vi "Get Metadata.vi"(7 "error in":errorcluster, 9 "measurement control path":path, 10 "measurement plugin service in":refnum<class "Measurement Plugin Service.lvclass">) -> (0 "error out":errorcluster, 2 "metadata value":T2(array[cluster]), 3 "measurement plugin service out":refnum<class "Measurement Plugin Service.lvclass">)   [LabVIEW 2020, in "Measurement Plugin Measurement Server.lvlib"]
uses:
  Measurement Plugin Measurement Server.lvlib
  TypeDefs/Parameter Annotations Entry.ctl
  Measurement Plugin Service/Measurement Plugin Service.lvclass
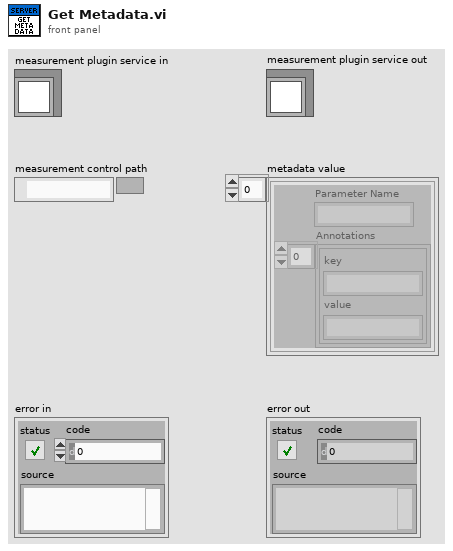
[diagram p1: front panel]
types:
  T1 = typedef "Measurement Plugin Measurement Server.lvlib/Parameter Annotations Entry.ctl" = cluster{"key":string, "value":string}
  T2 = cluster{"Parameter Name":string, "Annotations":T1[]}[]
  T3 = typedef "Measurement Plugin Measurement Server.lvlib/Parameter Type Specialization.ctl" = cluster{"parameter name":string, "type specialization":T4, "annotations":cluster{"key":T5, "value":string}[]}
  T4 = typedef "Measurement Plugin Measurement Server.lvlib/Type Specialization.ctl" = enum16{"none", "pin", "path", "enum", "ioresource"}
  T5 = typedef "Measurement Plugin Measurement Server.lvlib/Type Specialization Key.ctl" = enum16{"none", "pin.instrument_type", "enum.values", "ioresource.instrument_type"}
  T6 = cluster{"Parameter Name":string, "Annotations":T1[]}
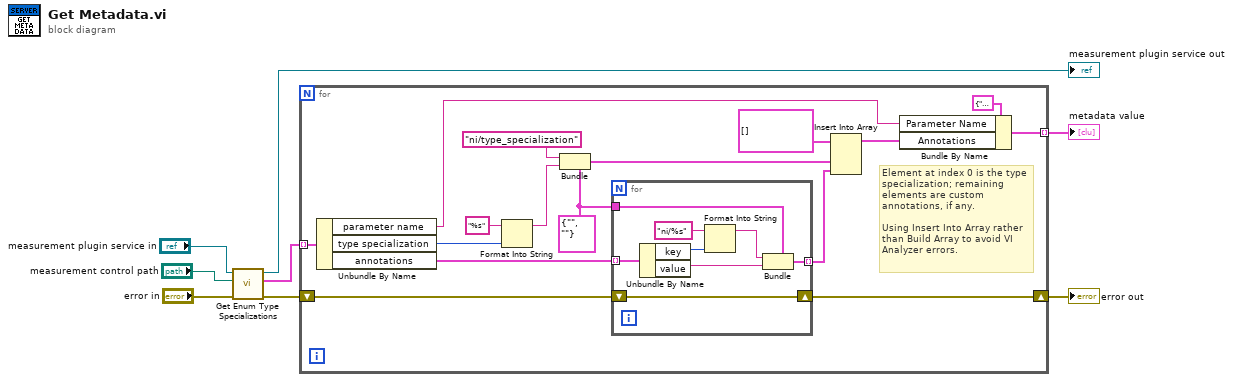
[diagram p0: block diagram]
diagram:
  n1 = call "Get Enum Type Specializations.vi"("error in"="error in", "measurement control path"="measurement control path", "measurement plugin service in"="measurement plugin service in") -> ("error out"=w5:errorcluster, "type specializations"=w6:T3[], "measurement plugin service out"=→"measurement plugin service out":refnum<class "Measurement Plugin Service.lvclass">)  [unwired: 6 in]
  n2 = for {
    tunnel: w6 -> [w24] mode=indexing
    shift-right: [w20] -> w7
    shift-left: w5 -> [w21]
    tunnel: [w22] -> w8 mode=indexing
    w13 = T1 {"key"="", "value"=""} ("Parameter_AnnotationsEntry")
    # "Element at index 0 is the type specialization; remaining elements are custom annotations, if any.\n\nUsing Insert Into Array rather than Build Array to avoid VI Analyzer errors."
    n3 = Unbundle By Name(w24) -> ("parameter name"=w15:string, "type specialization"=w19:T4, "annotations"=w14:cluster{"key":T5, "value":string}[])
    n4 = Format Into String(format string="%s", w19) -> (resulting string=w17:string)  [unwired: 2 in, 1 out]
    n5 = Bundle(cluster=w13, "key"="ni/type_specialization" ("Value"), "value"=w17) -> (w12:T1)
    n6 = for {
      shift-right: [w32] -> w20
      shift-left: w21 -> [w32]
      tunnel: w14 -> [w31] mode=indexing
      tunnel: w13 -> [w26]
      tunnel: [w25] -> w11 mode=indexing
      n7 = Unbundle By Name(w31) -> ("key"=w29:T5, "value"=w27:string)
      n8 = Format Into String(format string="ni/%s", w29) -> (resulting string=w28:string)  [unwired: 2 in, 1 out]
      n9 = Bundle(cluster=w26, "key"=w28, "value"=w27) -> (w25:T1)
    }
    n10 = Insert Into Array(array=T1[] [], new element #1=w12, new element #2=w11) -> (w10:T1[])  [unwired: 1 in]
    n11 = Bundle By Name(cluster=T6 {"Parameter Name"="", "Annotations"=[{"key"="", "value"=""}]} ("Cluster"), "Parameter Name"=w15, "Annotations"=w10) -> (w22:T6)
  }
  "error out" <- w7
  "metadata value" <- w8
